vi "ManageDAQ.vi"(8 "error in":errorcluster, 9 "StreamTypeDef":T1, 10 "data type":variant) -> (0 "error out":errorcluster, 1 "StreamTypeDef":T1)   [LabVIEW 2024]
uses:
  Control/StreamTypeDef.ctl
  Control/streamIO_states.ctl
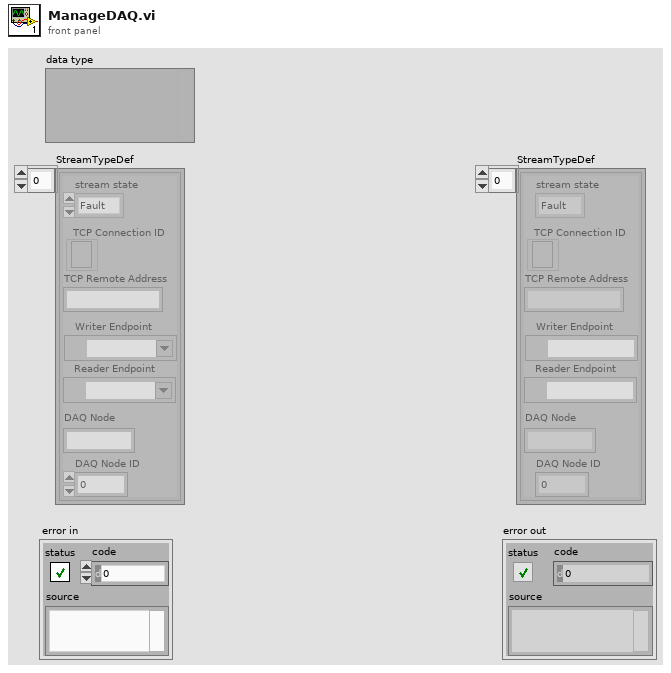
[diagram p1: front panel]
types:
  T1 = typedef "StreamTypeDef.ctl" = cluster{"stream state":T2, "TCP Remote Address":string, "TCP Connection ID":refnum<k5>, "Reader Endpoint":refnum<k21>, "Writer Endpoint":refnum<k21>, "DAQ Node":string, "DAQ Node ID":i32}[]
  T2 = typedef "streamIO_states.ctl" = enum16{"Fault", "Initilize", "Stream", "Close"}
  T3 = enum16{"Standard", "Buffered", "CRLF", "Immediate"}
  T4 = cluster{"stream state":T2, "TCP Remote Address":string, "TCP Connection ID":refnum<k5>, "Reader Endpoint":refnum<k21>, "Writer Endpoint":refnum<k21>, "DAQ Node":string, "DAQ Node ID":i32}
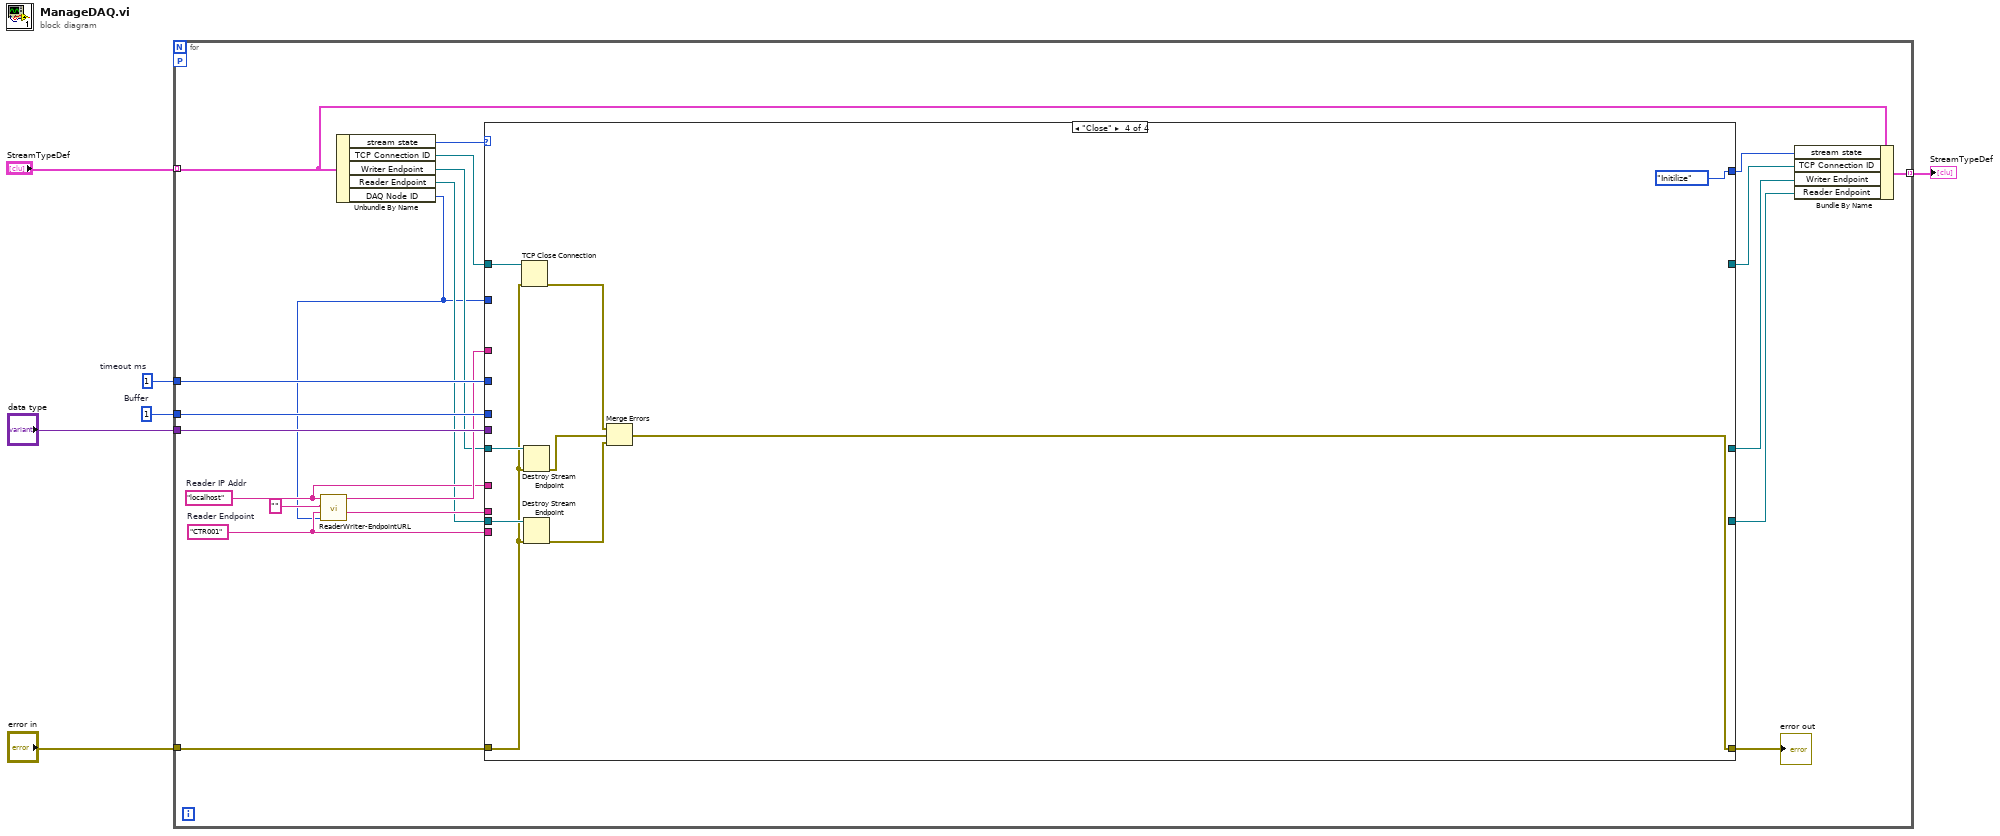
[diagram p0: block diagram]
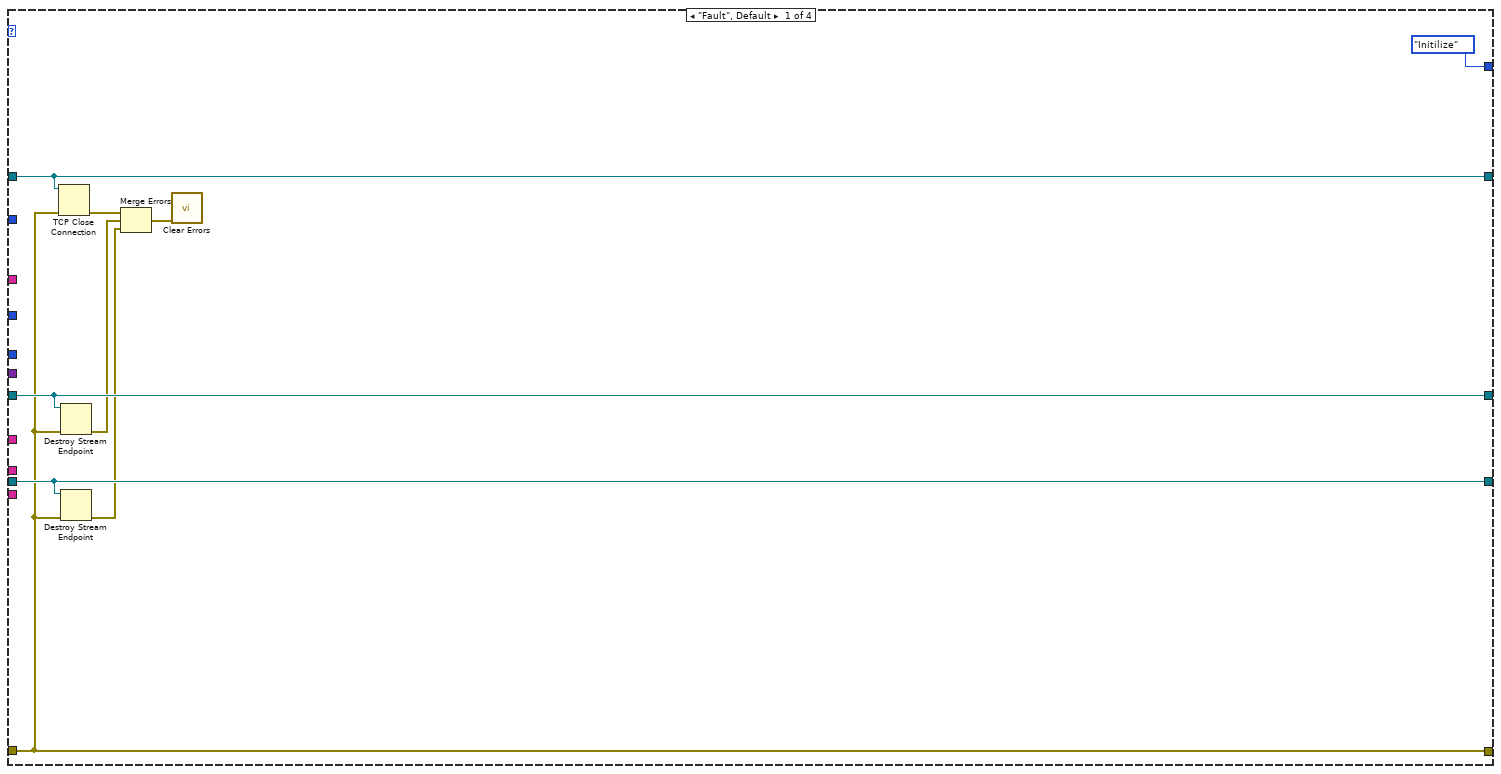
[diagram p2: hidden frame]
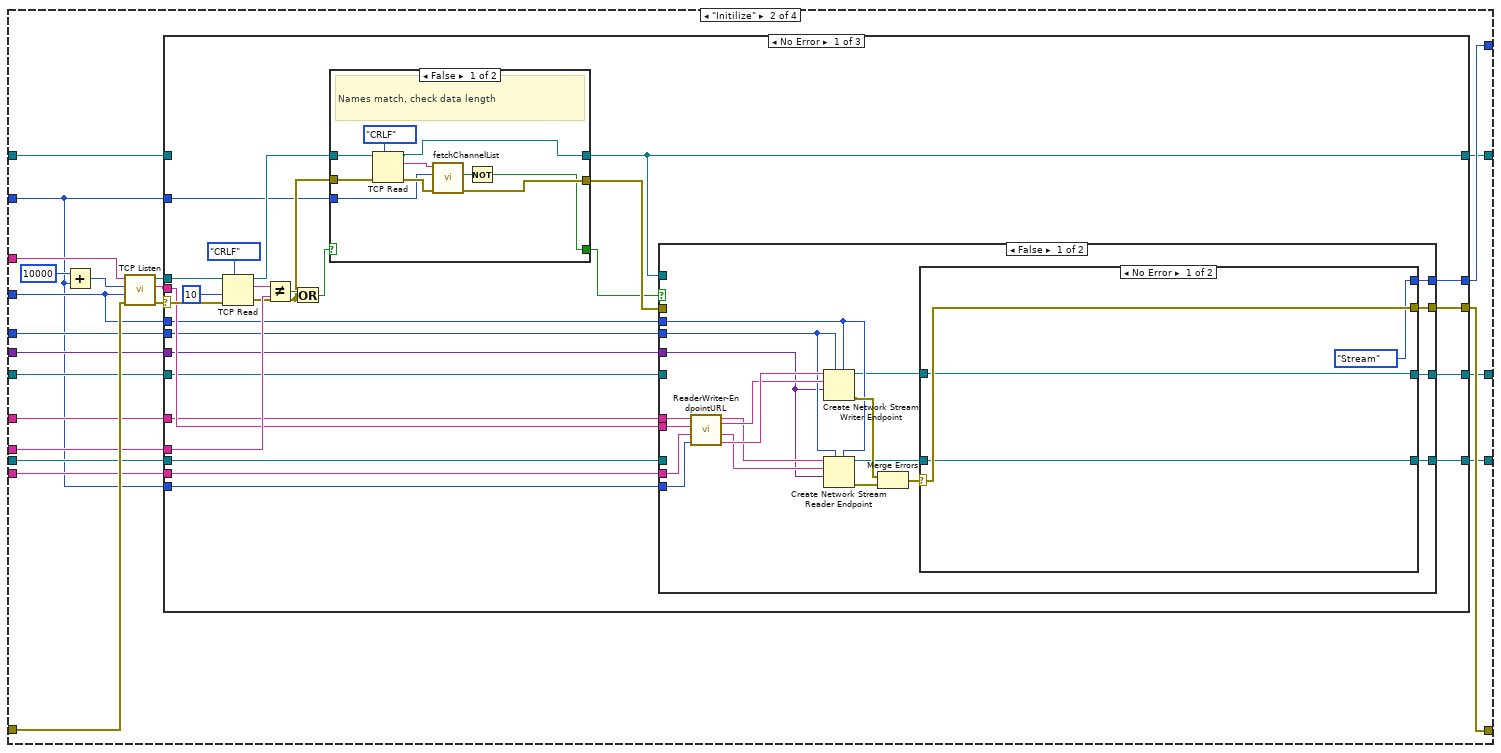
[diagram p3: hidden frame]
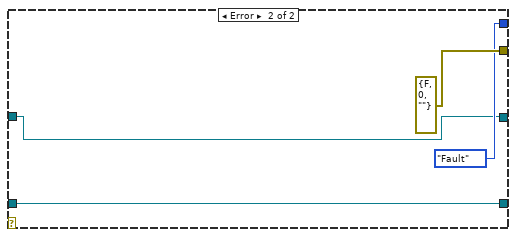
[diagram p5: hidden frame]
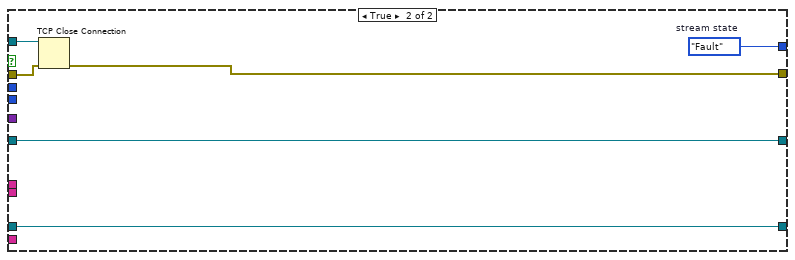
[diagram p6: hidden frame]
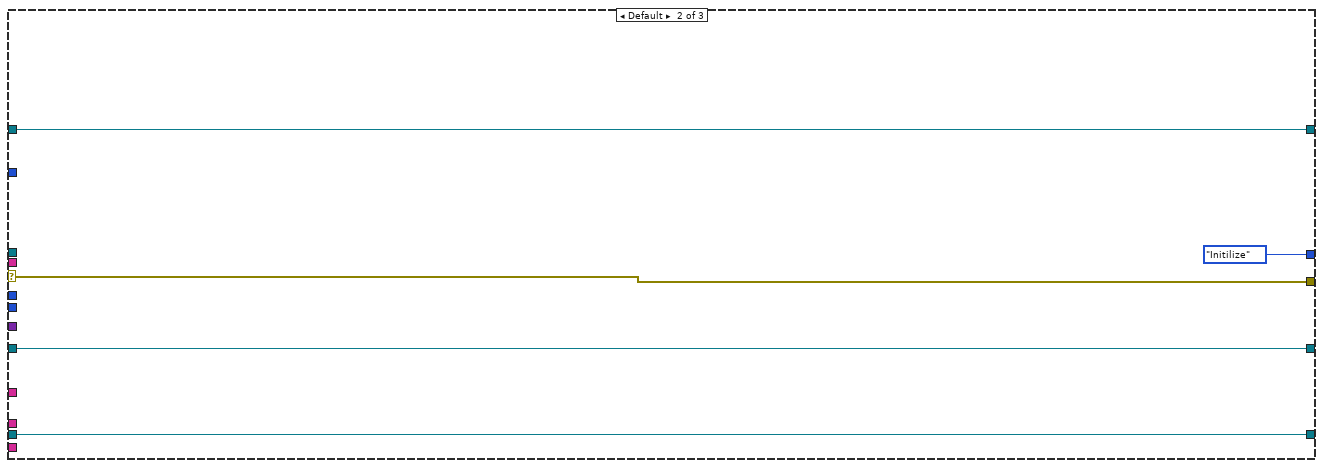
[diagram p7: hidden frame]
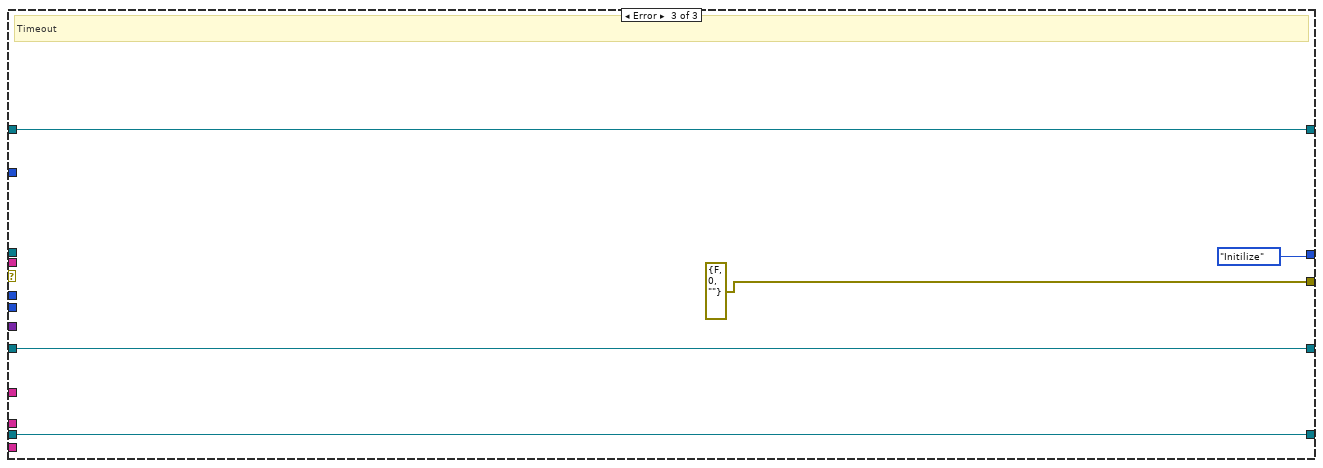
[diagram p8: hidden frame]
diagram:
  w4 = 1  # Buffer
  w5 = 1  # timeout ms
  n1 = for {
    tunnel: "error in" -> [w27]
    tunnel: w5 -> [w26]
    tunnel: w4 -> [w25]
    tunnel: "data type" -> [w24]
    tunnel: [w9] -> w1 mode=indexing
    tunnel: "StreamTypeDef" -> [w8] mode=indexing
    workers-P: _ -> [_]
    w21 = "localhost"  # Reader IP Addr
    w20 = "CTR001"  # Reader Endpoint
    n2 = Unbundle By Name(w8) -> ("stream state"=w19:T2, "TCP Connection ID"=w14:refnum<k5>, "Writer Endpoint"=w11:refnum<k21>, "Reader Endpoint"=w10:refnum<k21>, "DAQ Node ID"=w7:i32)
    n3 = call "ReaderWriter-EndpointURL.vi"("DAQ ID #"=w7, "CTR Endpoint"=w20, "DAQ IR Addr"="", "CTR IP Addr"=w21) -> ("DAQ Endpoint"=w22:string, "CTR URL"=w23:string)  [unwired: 4 in, 2 out]
    n4 = case shown="\"Close\"" w19 {
      selector: w19 -> [_ _ w143 _]
      tunnel: [streamIO_states."Initilize" ("Enum") w50 w143 streamIO_states."Initilize" ("Enum")] -> w18
      tunnel: w27 -> [w33 w58 w144 w149]
      tunnel: w26 -> [_ w45 _ _]
      tunnel: [w33 w56 w144 w145] -> w16
      tunnel: w23 -> [_ w55 _ _]
      tunnel: w22 -> [_ w51 _ _]
      tunnel: w21 -> [_ w48 _ _]
      tunnel: w20 -> [_ w47 _ _]
      tunnel: w25 -> [_ w46 _ _]
      tunnel: w24 -> [_ w44 _ _]
      tunnel: [w32 w43 _ _] -> w15
      tunnel: w14 -> [w32 w42 _ w150]
      tunnel: [w34 w41 _ _] -> w12
      tunnel: [w35 w40 _ _] -> w13
      tunnel: w11 -> [w34 w39 _ w151]
      tunnel: w10 -> [w35 w38 _ w152]
      tunnel: w7 -> [_ w37 _ _]
      frame "Fault", Default {
        n5 = TCP Close Connection(connection ID=w32, error in (no error)=w33) -> (error out=w31:errorcluster)  [unwired: 1 in, 1 out]
        n6 = Destroy Stream Endpoint(8:w33, 11:w34) -> (0:w30:errorcluster)
        n7 = Destroy Stream Endpoint(8:w33, 11:w35) -> (0:w29:errorcluster)
        n8 = Merge Errors(w31, w30, w29) -> (w28:errorcluster)
        n9 = call <vilib>:"Clear Errors.vi"("error in (no error)"=w28) -> ()  [unwired: 5 in, 2 out]
      }
      frame "Initilize" {
        n10 = Add(x=u16 10000 ("port"), y=w37) -> (x+y=w53:i32)
        n11 = call <vilib>:"TCP Listen.vi"("error in (no error)"=w58, "timeout ms (wait forever: -1)"=w45, "port"=w53, "service name"=w55) -> ("error out"=w57:errorcluster, "remote address"=w49:string, "connection ID"=w52:refnum<k5>)  [unwired: 3 in, 2 out]
        n12 = case shown="No Error" w57 {
          selector: w57 -> [w84 w137 _]
          tunnel: [w78 w137 errorcluster {"status"=FALSE, "code"=0, "source"=""} ("error IO")] -> w56
          tunnel: w52 -> [w83 _ _]
          tunnel: w51 -> [w81 _ _]
          tunnel: [w77 streamIO_states."Initilize" ("stream state") streamIO_states."Initilize" ("stream state")] -> w50
          tunnel: w49 -> [w76 _ _]
          tunnel: w48 -> [w75 _ _]
          tunnel: w47 -> [w74 _ _]
          tunnel: w37 -> [w73 _ _]
          tunnel: w46 -> [w72 _ _]
          tunnel: w45 -> [w71 _ _]
          tunnel: w44 -> [w70 _ _]
          tunnel: w37 -> [w64 _ _]
          tunnel: [w63 w135 w140] -> w43
          tunnel: w42 -> [_ w135 w140]
          tunnel: [w62 w134 w139] -> w41
          tunnel: [w61 w133 w138] -> w40
          tunnel: w39 -> [w60 w134 w139]
          tunnel: w38 -> [w59 w133 w138]
          frame No Error {
            n13 = TCP Read(connection ID=w83, error in (no error)=w84, 7:T3."CRLF" ("mode (standard)"), 9:10 ("timeout ms (25000)")) -> (connection ID out=w68:refnum<k5>, data out=w80:string, error out=w67:errorcluster)  [unwired: 1 in]
            n14 = Not Equal?(x=w80, y=w81) -> (x != y?=w79:bool)
            n15 = Or(x=w79, y=w67) -> (x .or. y?=w69:bool)
            n16 = case shown="False" w69 {
              selector: w69 -> [_ w98]
              tunnel: [w87 w98] -> w65
              tunnel: w68 -> [w95 w97]
              tunnel: [w86 w97] -> w63
              tunnel: w67 -> [w94 w96]
              tunnel: [w91 w96] -> w66
              tunnel: w64 -> [w89 _]
              frame False {
                # "Names match, check data length"
                n17 = TCP Read(connection ID=w95, error in (no error)=w94, 7:T3."CRLF" ("mode (standard)")) -> (connection ID out=w86:refnum<k5>, data out=w90:string, error out=w92:errorcluster)  [unwired: 2 in]
                n18 = call "fetchChannelList.vi"("error in"=w92, "DAQ ID #"=w89, "Channels"=w90) -> ("error out"=w91:errorcluster, "Channel Match?"=w88:bool)  [unwired: 6 in, 1 out]
                n19 = Not(x=w88) -> (.not. x?=w87:bool)
              }
              frame True {
                # "names not equal, abort"
              }
            }
            n20 = case shown="False" w65 {
              tunnel: w63 -> [_ w132]
              tunnel: w66 -> [_ w131]
              tunnel: [w115 w130] -> w78
              tunnel: [w114 w129] -> w77
              tunnel: w76 -> [w113 _]
              tunnel: w75 -> [w112 _]
              tunnel: w74 -> [w111 _]
              tunnel: w73 -> [w110 _]
              tunnel: w72 -> [w105 _]
              tunnel: w71 -> [w104 _]
              tunnel: w70 -> [w103 _]
              tunnel: [w101 w128] -> w62
              tunnel: [w100 w127] -> w61
              tunnel: w60 -> [_ w128]
              tunnel: w59 -> [_ w127]
              frame False {
                n21 = call "ReaderWriter-EndpointURL.vi"("DAQ ID #"=w110, "CTR Endpoint"=w111, "DAQ IR Addr"=w113, "CTR IP Addr"=w112) -> ("CTR Endpoint"=w109:string, "DAQ Endpoint"=w106:string, "DAQ URL"=w108:string, "CTR URL"=w107:string)  [unwired: 4 in]
                n22 = Create Network Stream Writer Endpoint(5:w104, 7:w105, 9:w103, 10:w108, 11:w109) -> (0:w116:errorcluster, 3:w102:refnum<k21>)  [unwired: 2 in]
                n23 = Create Network Stream Reader Endpoint(5:w104, 7:w105, 9:w103, 10:w106, 11:w107) -> (0:w117:errorcluster, 3:w99:refnum<k21>)  [unwired: 2 in]
                n24 = Merge Errors(w116, w117) -> (w118:errorcluster)
                n25 = case shown="No Error" w118 {
                  selector: w118 -> [w122 _]
                  tunnel: [w122 errorcluster {"status"=FALSE, "code"=0, "source"=""} ("error IO")] -> w115
                  tunnel: [streamIO_states."Stream" ("stream state") streamIO_states."Fault" ("stream state")] -> w114
                  tunnel: [w120 w124] -> w101
                  tunnel: w102 -> [w120 w124]
                  tunnel: [w119 w123] -> w100
                  tunnel: w99 -> [w119 w123]
                  frame No Error {
                  }
                  frame Error {
                  }
                }
              }
              frame True {
                w129 = streamIO_states."Fault"  # stream state
                n26 = TCP Close Connection(connection ID=w132, error in (no error)=w131) -> (error out=w130:errorcluster)  [unwired: 1 in, 1 out]
              }
            }
          }
          frame Default {
          }
          frame Error {
            # "Timeout"
          }
        }
      }
      frame "Stream" {
      }
      frame "Close" {
        n27 = TCP Close Connection(connection ID=w150, error in (no error)=w149) -> (error out=w146:errorcluster)  [unwired: 1 in, 1 out]
        n28 = Destroy Stream Endpoint(8:w149, 11:w151) -> (0:w147:errorcluster)
        n29 = Destroy Stream Endpoint(8:w149, 11:w152) -> (0:w148:errorcluster)
        n30 = Merge Errors(w146, w147, w148) -> (w145:errorcluster)
      }
    }
    "error out" <- w16
    n31 = Bundle By Name(cluster=w8, "stream state"=w18, "TCP Connection ID"=w15, "Writer Endpoint"=w12, "Reader Endpoint"=w13) -> (w9:T4)
  }
  "StreamTypeDef" <- w1
